vi "LDO Trigger Events.vi"(0 "Event Booleans in":T1, 1 "Burner ON Ref":refnum<vi>, 2 "0.8 ML Ref":refnum<vi>, 3 "1.1 ML Ref":refnum<vi>, 4 "1.33 ML Ref":refnum<vi>, 7 "Oil spray 0.8cc/min - LDO":bool, 8 "Burner ON":bool, 9 "Oil spray 1.1cc/min - LDO":bool, 11 "Oil spray 1.33cc/min - LDO":bool) -> (14 "Event Booleans out":T1)   [LabVIEW 2020]
uses:
  Event Booleans.ctl
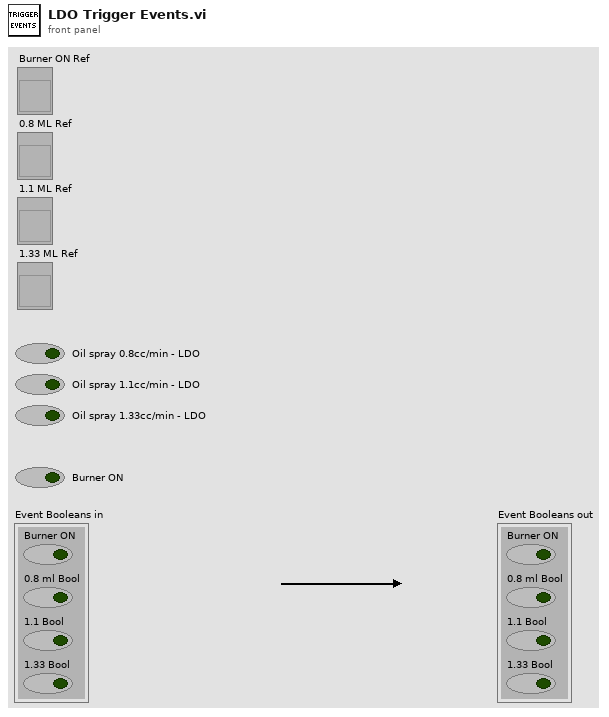
[diagram p1: front panel]
types:
  T1 = typedef "Event Booleans.ctl" = cluster{"Burner ON":bool, "0.8 ml Bool":bool, "1.1 Bool":bool, "1.33 Bool":bool}
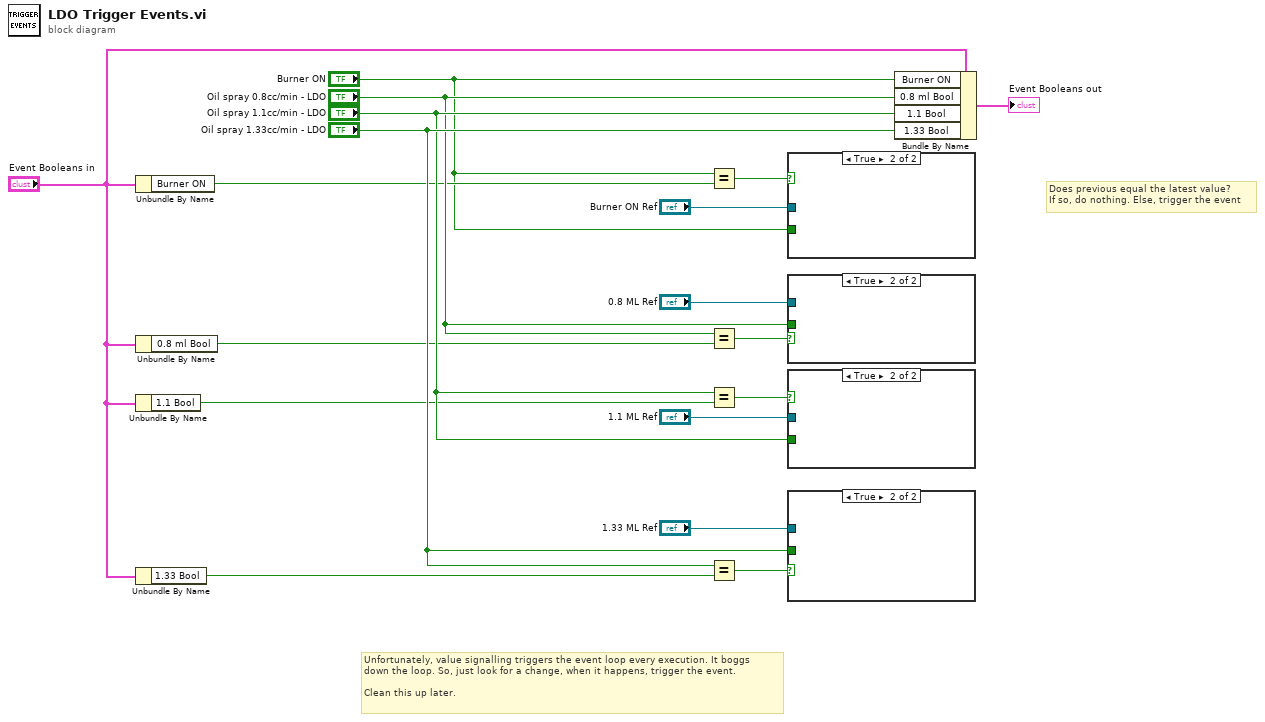
[diagram p0: block diagram]
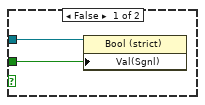
[diagram p2: hidden frame]
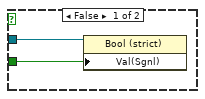
[diagram p3: hidden frame]
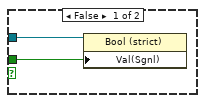
[diagram p4: hidden frame]
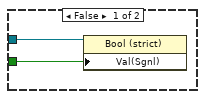
[diagram p5: hidden frame]
diagram:
  # "Does previous equal the latest value?\nIf so, do nothing. Else, trigger the event"
  # "Unfortunately, value signalling triggers the event loop every execution. It boggs\ndown the loop. So, just look for a change, when it happens, trigger the event. \n\nClean this up later."
  n1 = Unbundle By Name("Event Booleans in") -> ("Burner ON"=w6:bool)
  n2 = Unbundle By Name("Event Booleans in") -> ("0.8 ml Bool"=w5:bool)
  n3 = Unbundle By Name("Event Booleans in") -> ("1.1 Bool"=w4:bool)
  n4 = Unbundle By Name("Event Booleans in") -> ("1.33 Bool"=w2:bool)
  n5 = Equal?(x="Burner ON", y=w6) -> (x = y?=w11:bool)
  n6 = Equal?(x="Oil spray 0.8cc/min - LDO", y=w5) -> (x = y?=w13:bool)
  n7 = Equal?(x="Oil spray 1.1cc/min - LDO", y=w4) -> (x = y?=w15:bool)
  n8 = Equal?(x="Oil spray 1.33cc/min - LDO", y=w2) -> (x = y?=w14:bool)
  n9 = case shown="True" w11 {
    tunnel: "Burner ON" -> [w20 _]
    tunnel: "Burner ON Ref" -> [w19 _]
    frame False {
      n10 = property on="Property Node" class="Bool (strict)"(reference=w19, "Val(Sgnl)"=w20) -> ()  [unwired: 1 in, 2 out]
    }
    frame True {
    }
  }
  n11 = case shown="True" w13 {
    tunnel: "Oil spray 0.8cc/min - LDO" -> [w22 _]
    tunnel: "0.8 ML Ref" -> [w21 _]
    frame False {
      n12 = property on="Property Node" class="Bool (strict)"(reference=w21, "Val(Sgnl)"=w22) -> ()  [unwired: 1 in, 2 out]
    }
    frame True {
    }
  }
  n13 = case shown="True" w15 {
    tunnel: "Oil spray 1.1cc/min - LDO" -> [w24 _]
    tunnel: "1.1 ML Ref" -> [w23 _]
    frame False {
      n14 = property on="Property Node" class="Bool (strict)"(reference=w23, "Val(Sgnl)"=w24) -> ()  [unwired: 1 in, 2 out]
    }
    frame True {
    }
  }
  n15 = case shown="True" w14 {
    tunnel: "Oil spray 1.33cc/min - LDO" -> [w26 _]
    tunnel: "1.33 ML Ref" -> [w25 _]
    frame False {
      n16 = property on="Property Node" class="Bool (strict)"(reference=w25, "Val(Sgnl)"=w26) -> ()  [unwired: 1 in, 2 out]
    }
    frame True {
    }
  }
  n17 = Bundle By Name(cluster="Event Booleans in", "Burner ON"="Burner ON", "0.8 ml Bool"="Oil spray 0.8cc/min - LDO", "1.1 Bool"="Oil spray 1.1cc/min - LDO", "1.33 Bool"="Oil spray 1.33cc/min - LDO") -> (→"Event Booleans out":T1)
